vi "SPM.vi"(8 "Stopp":bool, 10 "SLOT":i32=100 min=0 max=999 step=100 format="%03d", 11 "USB":i32) -> ()   [LabVIEW 2020]
doc: "This VI provides a GUI for SPM modules. It implements an abstract module interface, where callers provide the only necessary and sufficient information for callee modules via the datafields USB, SLOT and Stopp. All module intern information are handled hidden by the module. Thereby, a caller must not \"know\" about such internals."
uses:
  <vilib>/Platform/TimedLoop/XDataNode/timing_clust.ctl
  <vilib>/Platform/TimedLoop/XDataNode/nitl_modes.ctl
  <vilib>/Platform/TimedLoop/XDataNode/wakeup.ctl
  <vilib>/platform/TimedLoop/XDataNode/XDataNode.xnode
  <vilib>/Platform/TimedLoop/XDataNode/XDNodeRunTimeDep.lvlib
panel:
  in  "Set Pump State":bool
  out "Pump State":bool
  in  "Set Pump Mode":bool
  out "Pump Mode":bool
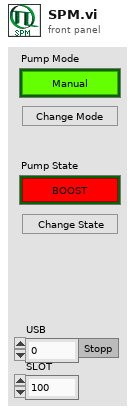
[diagram p1: front panel]
types:
  T1 = cluster{"PumpState":enum8{"BOOST", "ECO"}, "PumpMode":enum8{"static", "dynamic"}}
  T2 = typedef "XDNodeRunTimeDep.lvlib/timing_clust.ctl" = cluster{"Expected End [f-1]":u64, "Actual End [f-1]":u64, "Finished Late? [f-1]":bool, "Expected End [i-1]":u64, "Actual End [i-1]":u64, "Finished Late? [i-1]":bool, "Expected Start [i]":u64, "Actual Start [i]":u64, "Expected Start [f]":u64, "Actual Start [f]":u64, "Source Name":string, "Structure Name":string, "Period":i64, "Deadline":i64, "Offset":i64, "Start":i64, "Priority":i32, "Timeout":i32, "Mode":T3, "Wakeup Reason":T4, "Error":errorcluster, "Source Type":string, "Secondary Source Type":string, "Global End Time":u64, "Global Start Time":u64, "Frame Duration":u64, "Iteration Duration":u64, "Assigned CPU":i32, "I/O Scan Engine Mode":u32}
  T3 = typedef "XDNodeRunTimeDep.lvlib/nitl_modes.ctl" = enum32{"No Change", "Process missed periods, maintain original phase", "Discard missed periods, maintain original phase", "Process missed periods, ignore original phase", "Discard missed periods, ignore original phase"}
  T4 = typedef "XDNodeRunTimeDep.lvlib/wakeup.ctl" = enum32{"Normal", "Aborted", "Asynchronous wakeup", "Timing source error", "Timed loop error", "Timeout"}
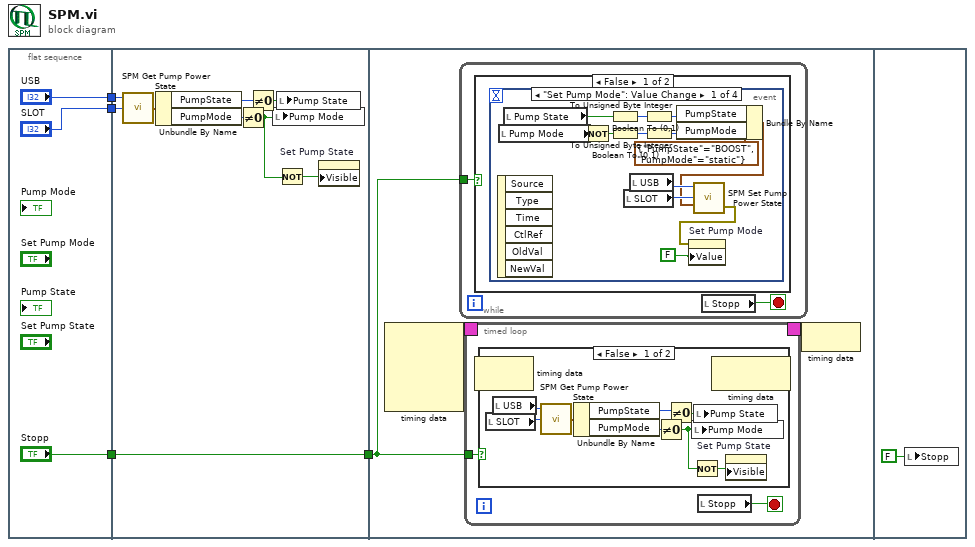
[diagram p0: block diagram]
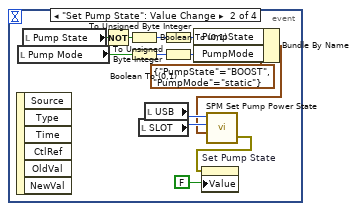
[diagram p2: hidden frame]
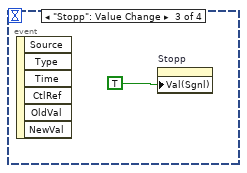
[diagram p3: hidden frame]
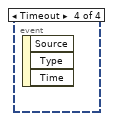
[diagram p4: hidden frame]
diagram:
  n1 = flat-sequence {
    tunnel: ["USB"] -> w4
    tunnel: ["SLOT"] -> w3
    tunnel: ["Stopp"] -> w1
    tunnel: w4 -> [w16]
    tunnel: w3 -> [w15]
    tunnel: [w8] -> w2
    tunnel: w1 -> [w8]
    tunnel: w2 -> [w17]
    frame #0 {
    }
    frame #1 {
      n2 = call "SPM Get Pump Power State.vi"("SlotId"=w15, "DevIdx"=w16) -> ("Pump Power State"=w14:T1)  [unwired: 1 in, 2 out]
      n3 = Unbundle By Name(w14) -> ("PumpState"=w12:enum8{"BOOST", "ECO"}, "PumpMode"=w13:enum8{"static", "dynamic"})
      n4 = Not Equal To 0?(x=w13) -> (x != 0?=w9:bool)
      n5 = Not Equal To 0?(x=w12) -> (x != 0?=w11:bool)
      n6 = local write "Pump Mode"(w9) -> ()
      n7 = local write "Pump State"(w11) -> ()
      n8 = Not(x=w9) -> (.not. x?=w10:bool)
      n9 = property on="Set Pump State" class="Bool (strict)"("Visible"=w10) -> ()  [unwired: 2 in, 2 out]
    }
    frame #2 {
      n10 = node-c288() -> (w19:T2)  [unwired: 4 in]
      n11 = while {
        tunnel: w17 -> [w20]
        stop <- w21 stop-if-true
        n12 = case shown="False" w20 {
          frame False {
            n13 = event shown="[0] \"Set Pump Mode\": Value Change" {
              selector: _ -> [_ _ _ _]
              dyn-events: _ -> [_ _ _ _]
              timeout: _ -> [_ _ _ _]
              event "Set Pump Mode": Value Change {
                n14 = event-data() -> ()  [unwired: 1 in, 6 out]
                n15 = local read "Pump Mode"() -> (w32:bool)
                n16 = local read "Pump State"() -> (w29:bool)
                n17 = Not(x=w32) -> (.not. x?=w31:bool)
                n18 = Boolean To (0,1)(Boolean=w29) -> (0, 1=w28:i16)
                n19 = Boolean To (0,1)(Boolean=w31) -> (0, 1=w27:i16)
                n20 = local read "SLOT"() -> (w33:i32)
                n21 = local read "USB"() -> (w34:i32)
                n22 = To Unsigned Byte Integer(number=w28) -> (unsigned 8bit integer=w26:u8)
                n23 = To Unsigned Byte Integer(number=w27) -> (unsigned 8bit integer=w23:u8)
                n24 = Bundle By Name(cluster=T1 {"PumpState"=enum."BOOST", "PumpMode"=enum."static"} ("Pump Power State"), "PumpState"=w26, "PumpMode"=w23) -> (w30:T1)
                n25 = call "SPM Set Pump Power State.vi"("Pump Power State"=w30, "SlotId"=w33, "DevIdx"=w34) -> ("error out"=w24:errorcluster)  [unwired: 1 in, 1 out]
                n26 = property on="Set Pump Mode" class="Bool (strict)"(error in=w24, "Value"=FALSE ("Set Pump State")) -> ()  [unwired: 1 in, 2 out]
              }
              event "Set Pump State": Value Change {
                n27 = event-data() -> ()  [unwired: 1 in, 6 out]
                n28 = local read "Pump Mode"() -> (w40:bool)
                n29 = local read "Pump State"() -> (w38:bool)
                n30 = Not(x=w38) -> (.not. x?=w39:bool)
                n31 = Boolean To (0,1)(Boolean=w39) -> (0, 1=w44:i16)
                n32 = Boolean To (0,1)(Boolean=w40) -> (0, 1=w43:i16)
                n33 = local read "SLOT"() -> (w46:i32)
                n34 = local read "USB"() -> (w47:i32)
                n35 = To Unsigned Byte Integer(number=w44) -> (unsigned 8bit integer=w41:u8)
                n36 = To Unsigned Byte Integer(number=w43) -> (unsigned 8bit integer=w42:u8)
                n37 = Bundle By Name(cluster=T1 {"PumpState"=enum."BOOST", "PumpMode"=enum."static"} ("Pump Power State"), "PumpState"=w41, "PumpMode"=w42) -> (w45:T1)
                n38 = call "SPM Set Pump Power State.vi"("Pump Power State"=w45, "SlotId"=w46, "DevIdx"=w47) -> ("error out"=w35:errorcluster)  [unwired: 1 in, 1 out]
                n39 = property on="Set Pump State" class="Bool (strict)"(error in=w35, "Value"=FALSE ("Set Pump State")) -> ()  [unwired: 1 in, 2 out]
              }
              event "Stopp": Value Change {
                n40 = event-data() -> ()  [unwired: 1 in, 6 out]
                n41 = property on="Stopp" class="Bool (strict)"("Val(Sgnl)"=TRUE ("Value (Signaling)")) -> ()  [unwired: 2 in, 2 out]
              }
              event Timeout {
                n42 = event-data() -> ()  [unwired: 1 in, 3 out]
              }
            }
          }
          frame True {
          }
        }
        n43 = local read "Stopp"() -> (w21:bool)
      }
      n44 = timed-loop {
        timing: w19 -> [_]
        timing-out: [_] -> w18
        tunnel: w17 -> [w49]
        stop <- w50 stop-if-true
        n45 = node-c288() -> ()  [unwired: 1 in, 1 out]
        n46 = case shown="False" w49 {
          frame False {
            n47 = local read "SLOT"() -> (w54:i32)
            n48 = local read "USB"() -> (w55:i32)
            n49 = call "SPM Get Pump Power State.vi"("SlotId"=w54, "DevIdx"=w55) -> ("Pump Power State"=w53:T1)  [unwired: 1 in, 2 out]
            n50 = Unbundle By Name(w53) -> ("PumpState"=w57:enum8{"BOOST", "ECO"}, "PumpMode"=w58:enum8{"static", "dynamic"})
            n51 = Not Equal To 0?(x=w58) -> (x != 0?=w51:bool)
            n52 = Not Equal To 0?(x=w57) -> (x != 0?=w56:bool)
            n53 = local write "Pump Mode"(w51) -> ()
            n54 = Not(x=w51) -> (.not. x?=w52:bool)
            n55 = local write "Pump State"(w56) -> ()
            n56 = property on="Set Pump State" class="Bool (strict)"("Visible"=w52) -> ()  [unwired: 2 in, 2 out]
          }
          frame True {
          }
        }
        n57 = local read "Stopp"() -> (w50:bool)
        n58 = node-c288() -> ()  [unwired: 1 in, 1 out]
      }
      n59 = node-c288(w18) -> ()
    }
    frame #3 {
      n60 = local write "Stopp"(FALSE ("Stopp")) -> ()
    }
  }
